vi "LVIS_DcGlobals.vi"() -> ()   [LabVIEW 2015]
uses:
  Ctrls/LVIS_SAF Status.ctl
  Ctrls/LVIS_Msg State.ctl
panel:
  in  "EventLog":bool
  in  "RstrError":errorcluster
  in  "Overflow":bool
  in  "Msg State":T1
  in  "Disable":bool
  in  "Online":bool
  in  "LVIS Exit":bool
  in  "SAF State":T2 items=["Clear"=0, "SAF Active"=100, "SAF Complete"=101, "SAF > 50%"=102, "SAF < 50%"=103, "SAF Full"=104, "Unknown"=99]
  in  "General":T3
  in  "DataTransfer":T4
  in  "GetDateTime":T4
  in  "StatusPoll":T5
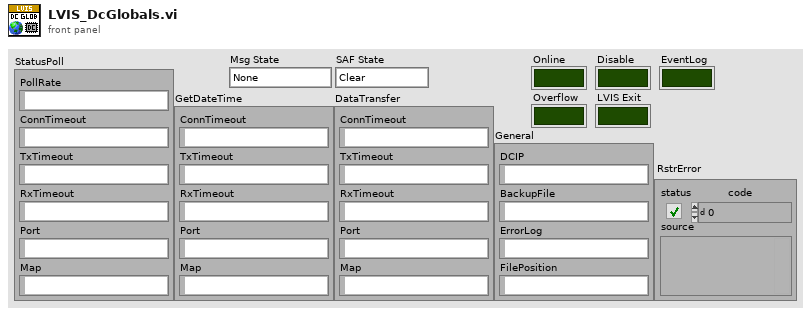
[diagram p1: front panel]
types:
  T1 = typedef "LVIS_Msg State.ctl" = enum16{"None", "Offline", "Online", "Backup Full"}
  T2 = typedef "LVIS_SAF Status.ctl" = u16
  T3 = cluster{"DCIP":string, "BackupFile":string, "ErrorLog":string, "FilePosition":string}
  T4 = cluster{"ConnTimeout":string, "TxTimeout":string, "RxTimeout":string, "Port":string, "Map":string}
  T5 = cluster{"PollRate":string, "ConnTimeout":string, "TxTimeout":string, "RxTimeout":string, "Port":string, "Map":string}
diagram:
